vi "XML Write Tubes.vi"(8 "error in":errorcluster, 11 "Tube Values":string[](array[string])) -> (0 "error out":errorcluster, 3 "File Saved":bool)   [LabVIEW 2023]
uses:
  TAGS.ctl
panel:
  out "Array":cluster{"TAG":T1}[][](array[cluster])
  in  "TAG":T1[](array[typedef])
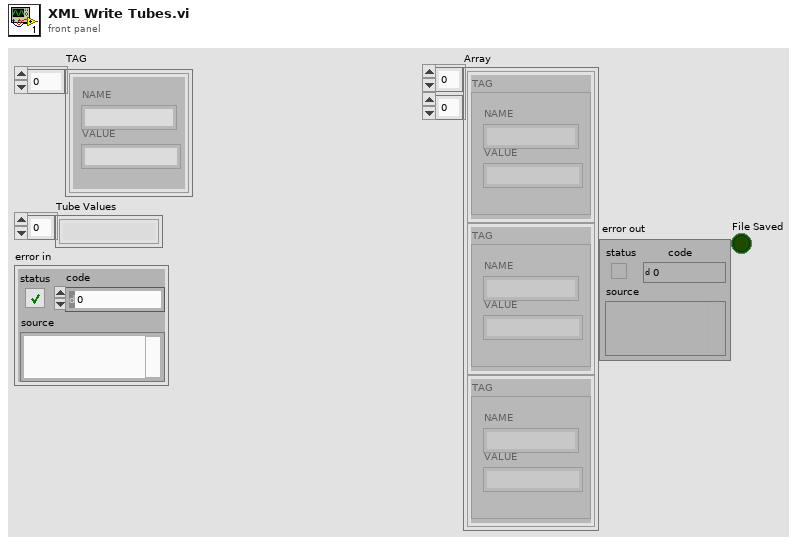
[diagram p1: front panel]
types:
  T1 = typedef "TAGS.ctl" = cluster{"NAME":string, "VALUE":string}
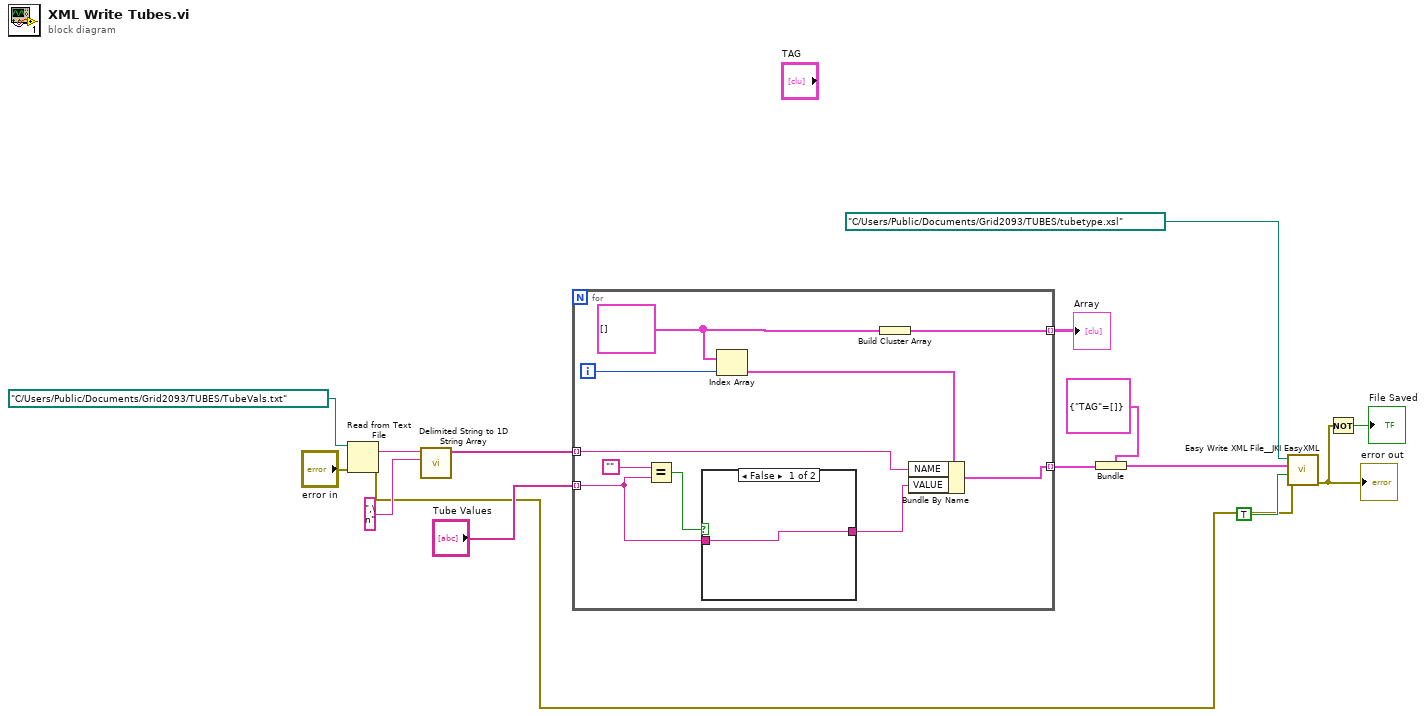
[diagram p0: block diagram]
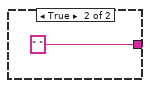
[diagram p2: hidden frame]
diagram:
  n1 = Read from Text File(file (use dialog)=path "C:/Users/Public/Documents/Grid2093/TUBES/TubeVals.txt" ("XML File Path"), error in="error in") -> (text=w6:string, error out=w1:errorcluster)  [unwired: 2 in, 2 out]
  n2 = call <vilib>:"Delimited String to 1D String Array.vi"("delimiter"=",\n", "delimited string"=w6) -> ("string array"=w4:string[])  [unwired: 9 in]
  n3 = for {
    tunnel: "Tube Values" -> [w16] mode=indexing
    tunnel: w4 -> [w21] mode=indexing
    tunnel: [w20] -> w12 mode=indexing
    tunnel: [w25] -> w14 mode=indexing
    i -> [w23]
    w24 = T1[] [] ("TAG")
    n4 = Equal?(x="", y=w16) -> (x = y?=w18:bool)
    n5 = case shown="False" w18 {
      tunnel: [w26 " "] -> w17
      tunnel: w16 -> [w26 _]
      frame False {
      }
      frame True {
      }
    }
    n6 = Index Array(array=w24, index=w23) -> (element=w22:T1)
    n7 = Build Cluster Array(w24) -> (w25:cluster{"TAG":T1}[])
    n8 = Bundle By Name(cluster=w22, "NAME"=w21, "VALUE"=w17) -> (w20:T1)
  }
  "Array" <- w14
  n9 = Bundle(cluster=cluster{"TAG":T1[]} {"TAG"=[]} ("TAGLIST"), "TAG"=w12) -> (w13:cluster{"TAG":T1[]})
  n10 = call <vilib>:"Easy Write XML File__JKI EasyXML.vi"("error in (no error)"=w1, "Overwrite File? (false)"=TRUE, "LabVIEW Data"=w13, "XML File Path"=path "C:/Users/Public/Documents/Grid2093/TUBES/tubetype.xsl") -> ("error out"=w8:errorcluster)  [unwired: 6 in, 1 out]
  "error out" <- w8
  n11 = Not(x=w8) -> (.not. x?=→"File Saved":bool)
